vi "SDCP SMF Receiver andTransmitter - Live Plot - Log File FGV.vi"(4 "error in (no error)":errorcluster, 5 "Command":enum16{"Initialize", "Acquire", "Save"}(ring), 6 "Trace file path":path, 7 "Raw frame":T1) -> (0 "error out":errorcluster)   [LabVIEW 2020]
uses:
  <vilib>/Utility/file.llb/Write Delimited Spreadsheet (string).vi
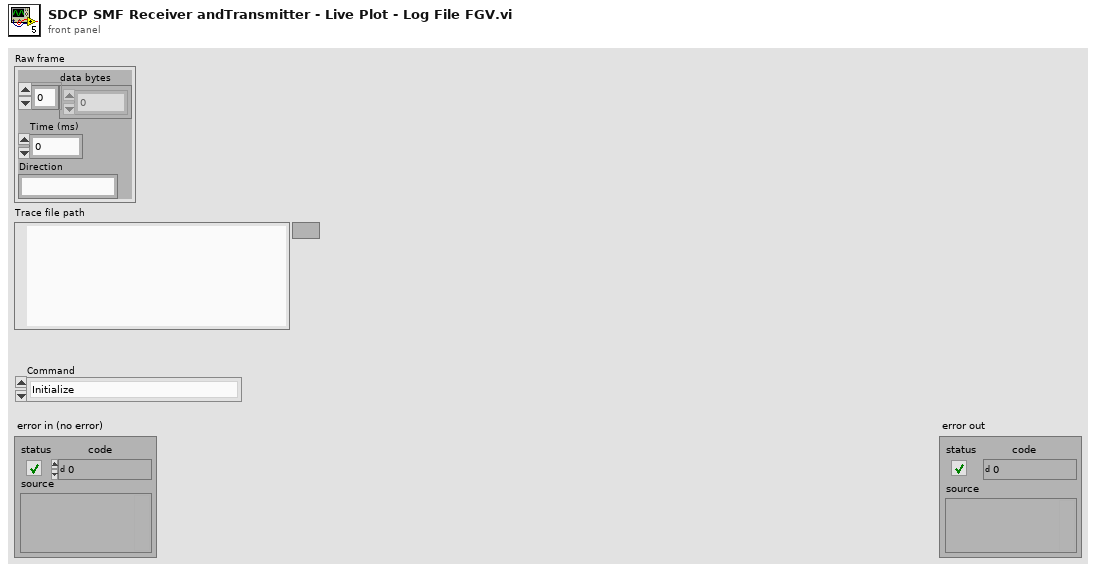
[diagram p1: front panel]
types:
  T1 = cluster{"data bytes":u8[], "Time (ms)":u32, "Direction":string}
  T2 = enum16{"open", "replace", "create", "open or create", "replace or create", "replace or create with confirmation"}
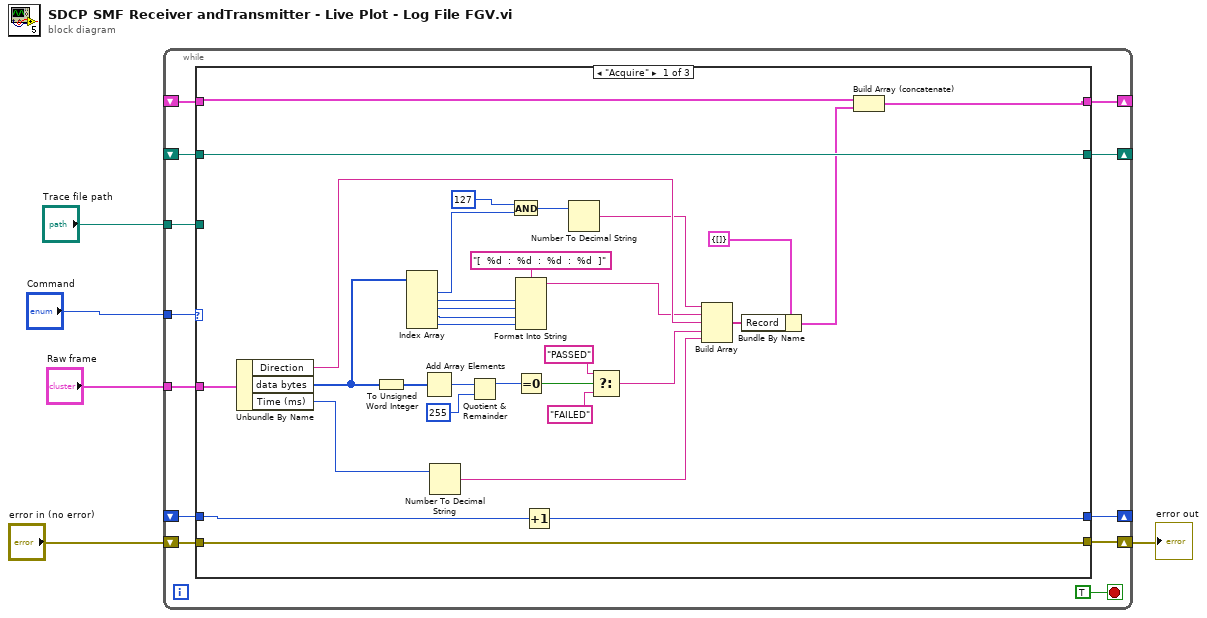
[diagram p0: block diagram]
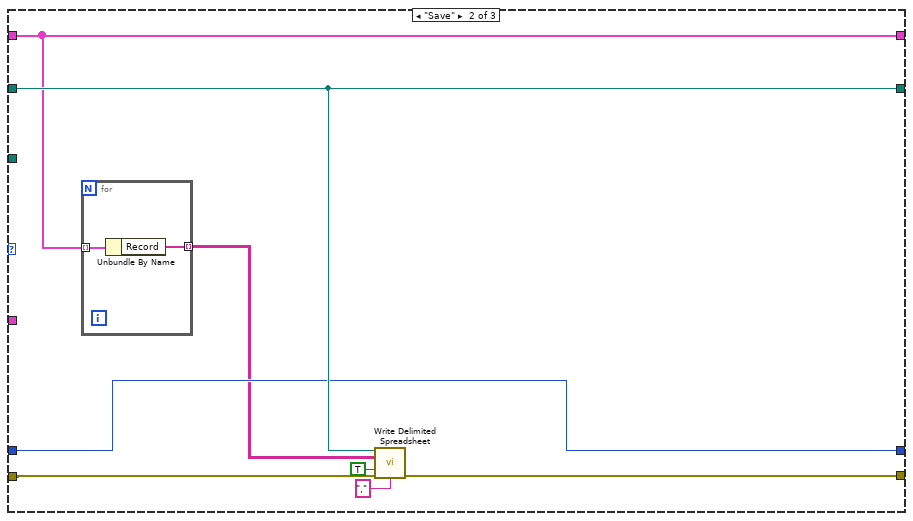
[diagram p2: hidden frame]
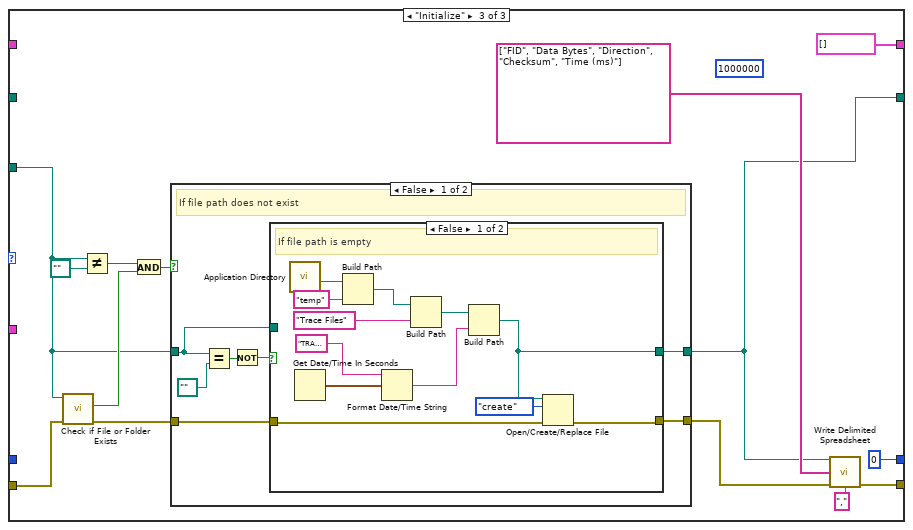
[diagram p3: hidden frame]
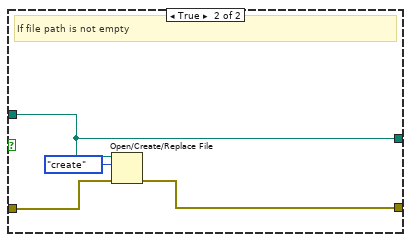
[diagram p4: hidden frame]
diagram:
  n1 = while {
    shift-right: [w11] -> w4
    shift-left: "error in (no error)" -> [w16]
    tunnel: "Command" -> [w15]
    shift-right: [w13] -> _
    shift-left: _ -> [w12]
    tunnel: "Trace file path" -> [w14]
    tunnel: "Raw frame" -> [w10]
    shift-right: [w8] -> _
    shift-left: _ -> [w9]
    shift-right: [w7] -> _
    shift-left: _ -> [w6]
    stop <- TRUE stop-if-true
    n2 = case shown="\"Acquire\"" w15 {
      tunnel: w16 -> [w25 w57 w73]
      tunnel: w14 -> [_ _ w65]
      tunnel: [w26 w56 w62] -> w13
      tunnel: w12 -> [w26 w56 _]
      tunnel: [w25 w55 w70] -> w11
      tunnel: w10 -> [w49 _ _]
      tunnel: w9 -> [w20 w51 _]
      tunnel: [w18 w51 cluster{"Record":string[]}[] []] -> w8
      tunnel: [w23 w52 0] -> w7
      tunnel: w6 -> [w24 w52 _]
      frame "Acquire" {
        n3 = Unbundle By Name(w49) -> ("Direction"=w32:string, "data bytes"=w43:u8[], "Time (ms)"=w33:u32)
        n4 = To Unsigned Word Integer(number=w43) -> (unsigned 16bit integer=w42:u16[])
        n5 = Index Array(array=w43) -> (element #1=w30:u8, element #2=w47:u8, element #3=w46:u8, element #4=w45:u8, element #5=w44:u8)  [unwired: 5 in]
        n6 = Add Array Elements(numeric array=w42) -> (sum=w41:u16)
        n7 = Number To Decimal String(number=w33) -> (decimal integer string=w35:string)  [unwired: 1 in]
        n8 = Quotient & Remainder(x=w41, y=u16 255) -> (x-y*floor(x/y)=w39:u16)  [unwired: 1 out]
        n9 = And(x=u8 127, y=w30) -> (x .and. y?=w28:u8)
        n10 = Format Into String(format string="[  %d  :  %d  :  %d  :  %d  ]", w47, w46, w45, w44) -> (resulting string=w31:string)  [unwired: 2 in, 1 out]
        n11 = Equal To 0?(x=w39) -> (x = 0?=w38:bool)
        n12 = Increment(x=w24) -> (x+1=w23:i32)
        n13 = Number To Decimal String(number=w28) -> (decimal integer string=w27:string)  [unwired: 1 in]
        n14 = Select(t="PASSED", s=w38, f="FAILED") -> (s? t:f=w34:string)
        n15 = Build Array(w27, w31, w32, w34, w35) -> (w21:string[])
        n16 = Bundle By Name(cluster=cluster{"Record":string[]} {"Record"=[]}, "Record"=w21) -> (w19:cluster{"Record":string[]})
        n17 = Build Array (concatenate)(w20, w19) -> (w18:cluster{"Record":string[]}[])
      }
      frame "Save" {
        n18 = for {
          tunnel: w51 -> [w59] mode=indexing
          tunnel: [w58] -> w50 mode=indexing
          n19 = Unbundle By Name(w59) -> ("Record"=w58:string[])
        }
        n20 = call-poly <vilib>:"Write Delimited Spreadsheet.vi"("file path (dialog if empty)"=w56, "2D data"=w50, "append to file? (new file:F)"=TRUE, "error in (no error)"=w57, "delimiter (\\t)"="," ("delimiter (\\t)")) -> ("error out"=w55:errorcluster)  [unwired: 9 in, 1 out]
      }
      frame "Initialize" {
        (unwired) 1000000 ("dimension size")
        n21 = call <vilib>:"Check if File or Folder Exists.vi"("error in (no error)"=w73, "path"=w65) -> ("error out"=w72:errorcluster, "file or folder exists?"=w66:bool)  [unwired: 7 in, 1 out]
        n22 = Not Equal?(x=w65, y=path "") -> (x != y?=w64:bool)
        n23 = And(x=w64, y=w66) -> (x .and. y?=w67:bool)
        n24 = case shown="False" w67 {
          tunnel: w72 -> [w80 w98]
          tunnel: w65 -> [w78 w97]
          tunnel: [w79 w98] -> w71
          tunnel: [w74 w97] -> w62
          frame False {
            # "If file path does not exist"
            n25 = Equal?(x=w78, y=path "") -> (x = y?=w76:bool)
            n26 = Not(x=w76) -> (.not. x?=w75:bool)
            n27 = case shown="False" w75 {
              tunnel: w80 -> [w84 w96]
              tunnel: w78 -> [_ w93]
              tunnel: [w83 w94] -> w79
              tunnel: [w82 w93] -> w74
              frame False {
                # "If file path is empty"
                n28 = call <vilib>:"Application Directory.vi"() -> ("Application Directory"=w92:path)
                n29 = Get Date/Time In Seconds() -> (seconds since 1Jan1904=w87:timestamp)
                n30 = Build Path(base path=w92, name or relative path="temp") -> (appended path=w90:path)
                n31 = Format Date/Time String(time format string (%c)="TRACE_%d_%m_%Y__%H_%M_%S.csv", seconds (now)=w87) -> (date/time string=w85:string)  [unwired: 1 in]
                n32 = Build Path(base path=w90, name or relative path="Trace Files") -> (appended path=w88:path)
                n33 = Build Path(base path=w88, name or relative path=w85) -> (appended path=w82:path)
                n34 = Open/Create/Replace File(file path (use dialog)=w82, error in=w84, operation (0:open)=T2."create") -> (error out=w83:errorcluster)  [unwired: 3 in, 2 out]
              }
              frame True {
                # "If file path is not empty"
                n35 = Open/Create/Replace File(file path (use dialog)=w93, error in=w96, operation (0:open)=T2."create") -> (error out=w94:errorcluster)  [unwired: 3 in, 2 out]
              }
            }
          }
          frame True {
            # "If file path exists"
          }
        }
        n36 = call-poly <vilib>:"Write Delimited Spreadsheet.vi"("file path (dialog if empty)"=w62, "1D data"=string[] ["FID", "Data Bytes", "Direction", "Checksum", "Time (ms)"], "error in (no error)"=w71, "delimiter (\\t)"="," ("delimiter (\\t)")) -> ("error out"=w70:errorcluster)  [unwired: 10 in, 1 out]
      }
    }
  }
  "error out" <- w4
